vi "Linear Temperature Image.vi"() -> ()   [LabVIEW 2015]
doc: "An example of how you can get different types of images from the camera.\n\nNOTE: You must have ThermoVision installed to run this example."
uses:
  <userlib>/ThermoVision/ThermoVision Digital.llb/ThermoVision Digital ImageType.ctl
  <vilib>/Analysis/Matrix/NI_Matrix.lvlib
  <vilib>/Analysis/Matrix/Numeric/Conversions/Matrix To Array - RM.vi
  <userlib>/ThermoVision/ThermoVision.llb/Thermovision CameraTypes.ctl
  <userlib>/ThermoVision/ThermoVision.llb/ThermoVision DeviceTypes.ctl
  <userlib>/ThermoVision/ThermoVision.llb/ThermoVision CommunicationInterfaceType.ctl
  <userlib>/ThermoVision/ThermoVision Digital.llb/ThermoVision Digital ImageMode.ctl
panel:
  in  "Height Down":bool
  in  "Height Up":bool
  in  "Width Down":bool
  in  "Width Up":bool
  in  "Box Down":bool
  in  "Box Right":bool
  in  "Box Left":bool
  in  "Box Up":bool
  out "Camera":T1(plugin-control)
  out "Kelvin Multiplier":dbl=10.0
  out "Celsius":dbl
  out "Height":dbl=80.0
  out "Width":dbl=80.0
  out "Measure Box Y":dbl
  out "Measure Box X":dbl
  out "Average":dbl
  out "Total":dbl
  out "Image(U16)":u16[][](array[numeric])
  in  "Image Mode":T2=enum."Temperature (0.1K)"
  in  "Interface":T3=enum."UVC"
  in  "Device":T4=enum."USB video"
  in  "Camera Serial Number":string
  in  "CameraType":T5=enum."FLIR A615/A645/SC645/SC655"
  in  "error in (no error)":errorcluster
  in  "Stop":bool
  out "error out":errorcluster
  # "Note:\n Before running this VI\n 1. Select camera type supporting \n      linear temperature image (A-series)\n 2. Type camera serial number, if you \n     have more than one firewire camera\n     connected.\n 3. Run the VI\n 4. Press Stop button to terminate \n     VI-execution"
  # "Box Width"
  # "Box Position"
  # "Box Height"
  # "Pre-run settings"
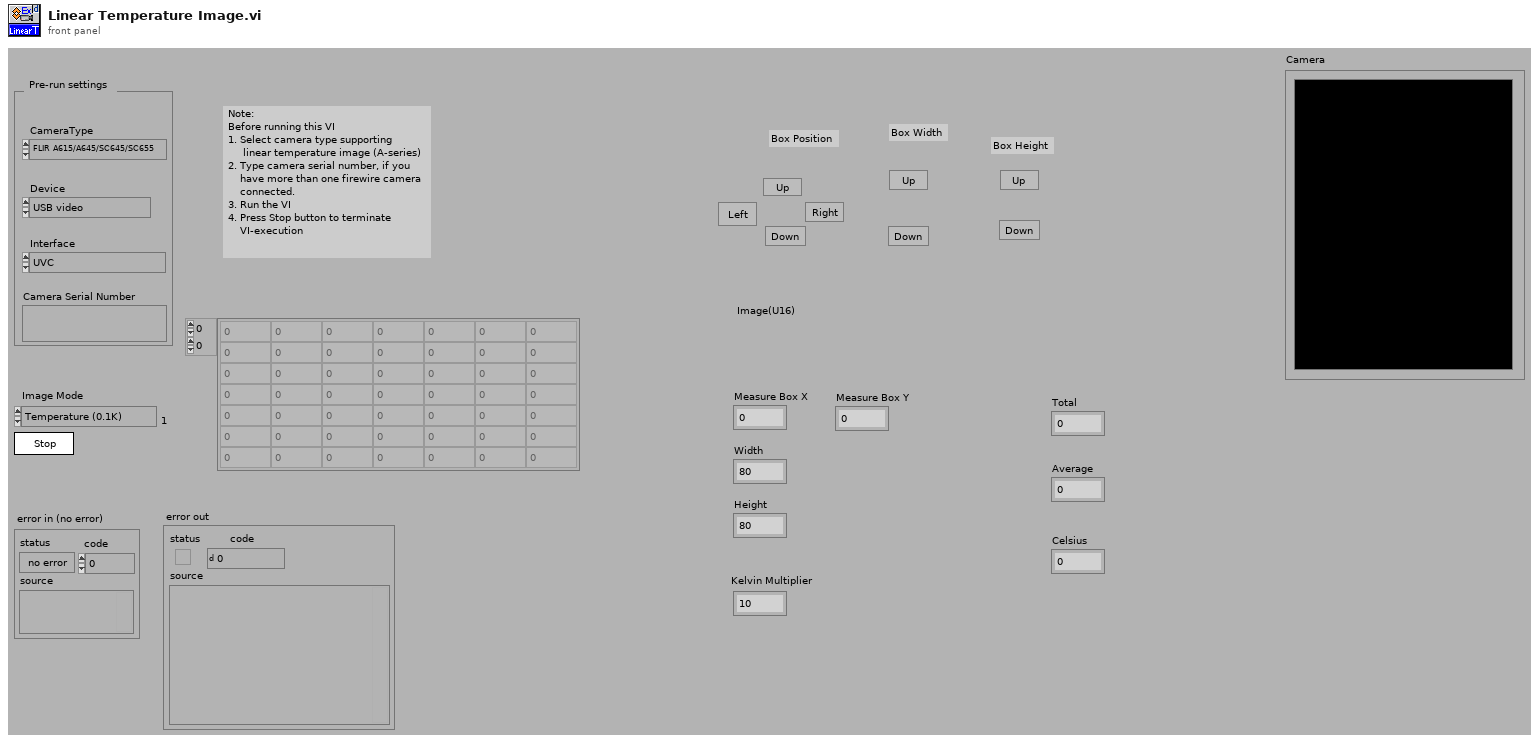
[diagram p1: front panel]
types:
  T1 = typedef "IMAQ Image.ctl" = refnum<image>
  T2 = typedef "ThermoVision Digital ImageMode.ctl" = enum16{"Signal", "Temperature (0.1K)", "Temperature (0.01K)"}
  T3 = typedef "ThermoVision CommunicationInterfaceType.ctl" = enum16{"File Only", "RS232", "TCP/IP(Ethernet)", "AV/C(FireWire)", "Gigabit Ethernet", "AXIS Video Server(Ethernet)", "UVC"}
  T4 = typedef "ThermoVision DeviceTypes.ctl" = enum16{"No Device", "FLIR PCCard", "ITEX IC-DIG 16", "Firewire 16-bit images", "Firewire 8-bit images", "Ethernet 16-bit images", "Ethernet 8-bit images", "IR-FlashLink", "iPort/GEV", "USB video"}
  T5 = typedef "Thermovision CameraTypes.ctl" = enum16{"ThermaCAM SC2000/SC3000", "THV 320/160", "ThermaCAM SC1000", "ThermaCAM S40/S45/S60/S65", "Thermovision A20/A40", "Cumulus SC4000/SC6000", "ThermaCAM SC640/SC660", "FLIR A320/A300/A310", "FLIR A325(A320G)/A315/SC305/SC325", "Indigo Merlin", "Indigo Phoenix", "Indigo Omega", "THV 1000", "THV 900", "FLIR GF320/GF309", "FLIR T-series", "FLIR A615/A645/SC645/SC655", "FLIR Exx series", "FLIR T620/T640/T420/T440"}
  T6 = enum16{"Internal Image Correction", "External Image Correction", "Auto Adjust", "Show Camera Info Dialog", "Show Device Status Dialog", "Reload Calibration(SC1000 only)"}
  T7 = enum16{"Unused0", "Unused1", "Unused2", "Unused3", "Unused4", "Unused5", "Unused6", "U16 Grayscale"}
  T8 = typedef "ThermoVision Digital ImageType.ctl" = enum16{"Raw", "Absolute", "Object", "Temperature", "Raw 8 bits"}
  T9 = typedef "Thermovision Object Reference.ctl" = refnum<k1>
  T10 = cluster{"Measure Box X":dbl, "Measure Box Y":dbl, dbl, dbl}
  T11 = typedef "LVPoint32TypeDef.ctl" = cluster{"Horizontal":i32, "Vertical":i32}
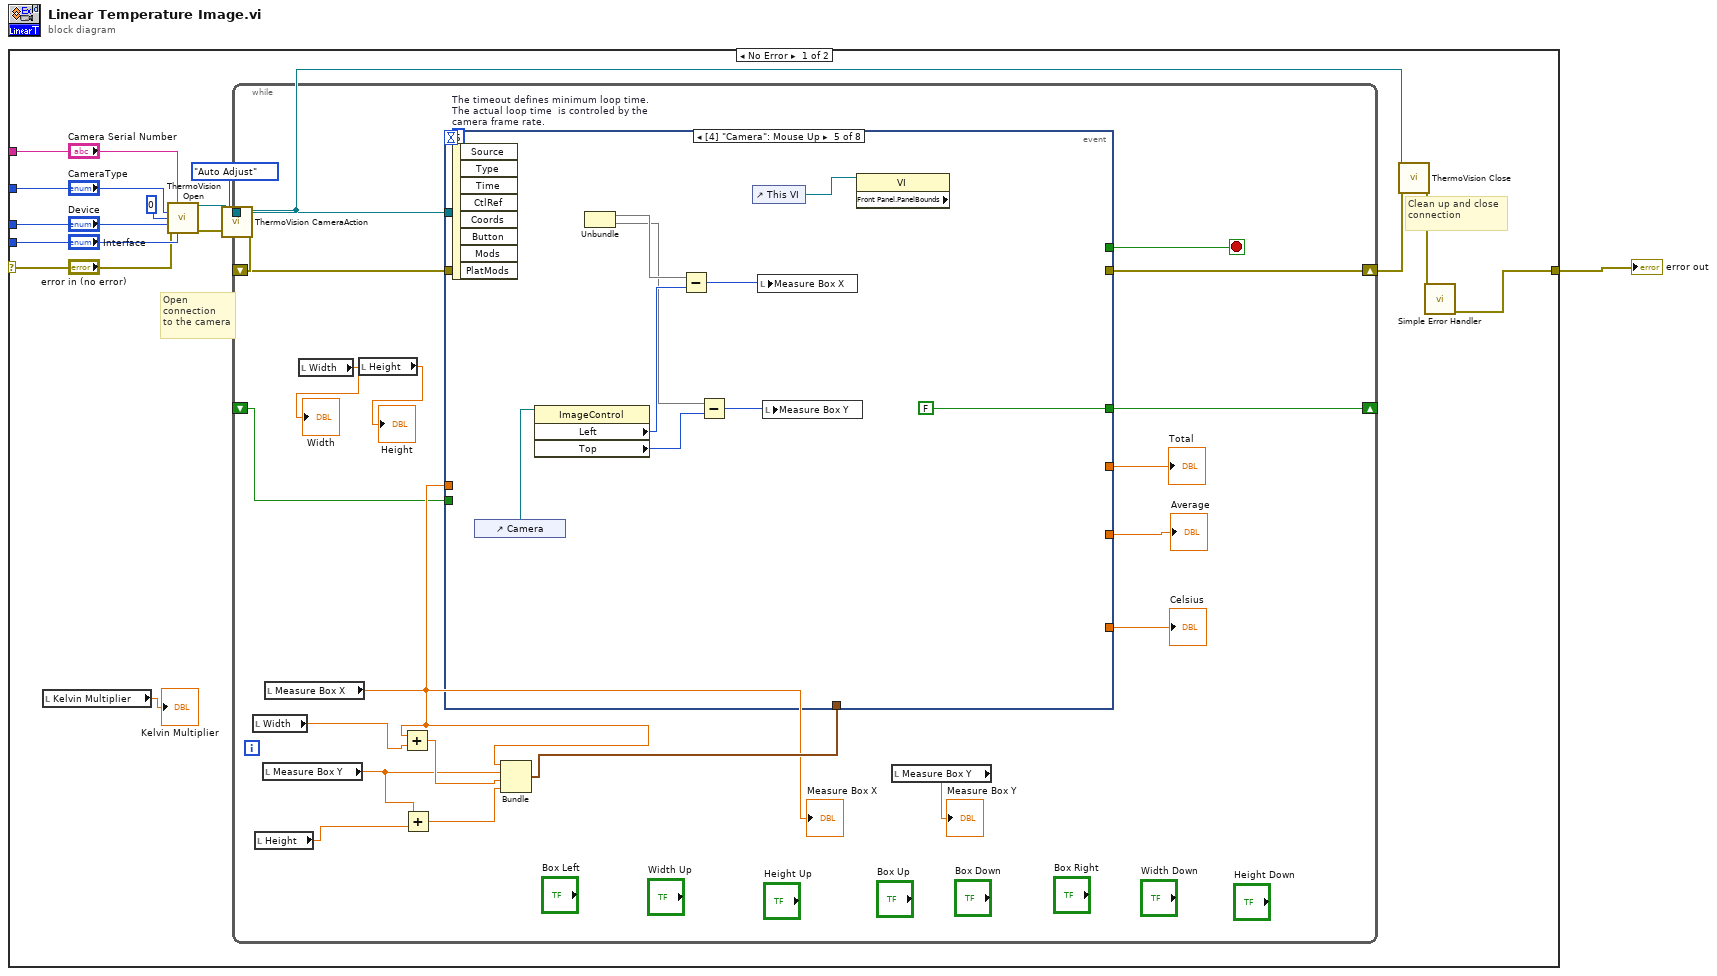
[diagram p0: block diagram]
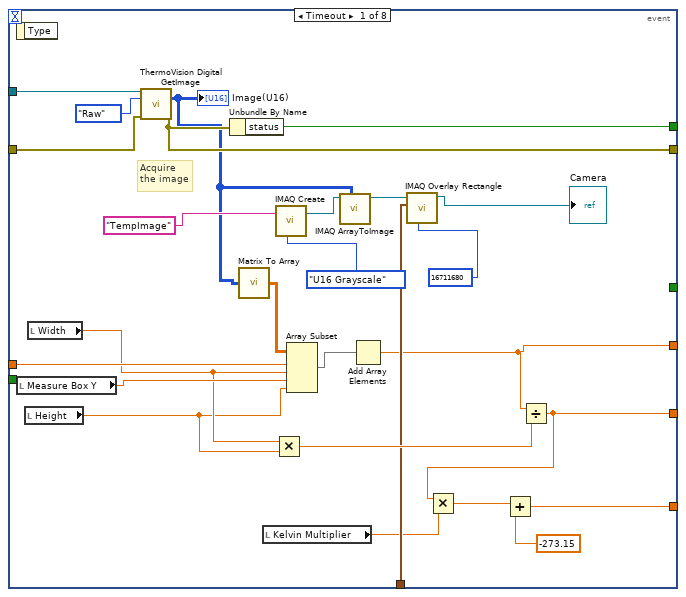
[diagram p2: hidden frame]
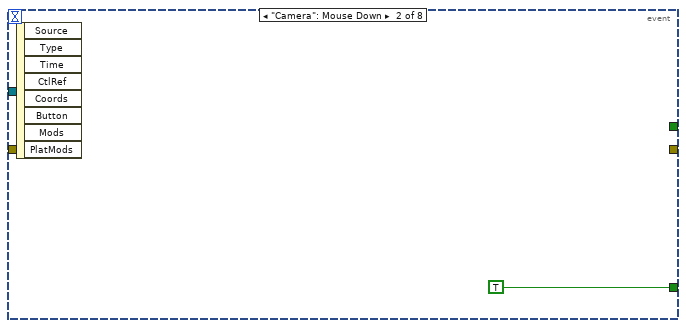
[diagram p3: hidden frame]
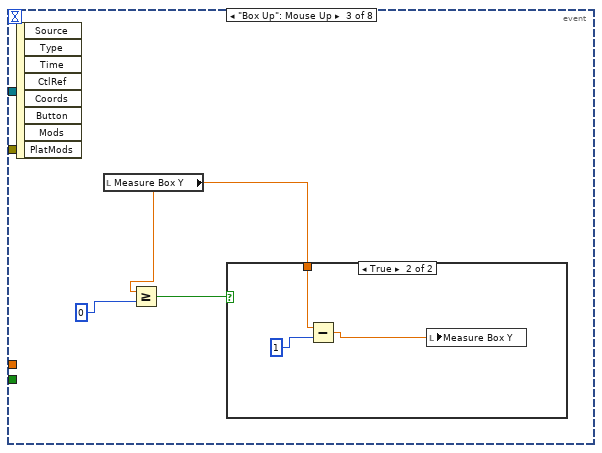
[diagram p4: hidden frame]
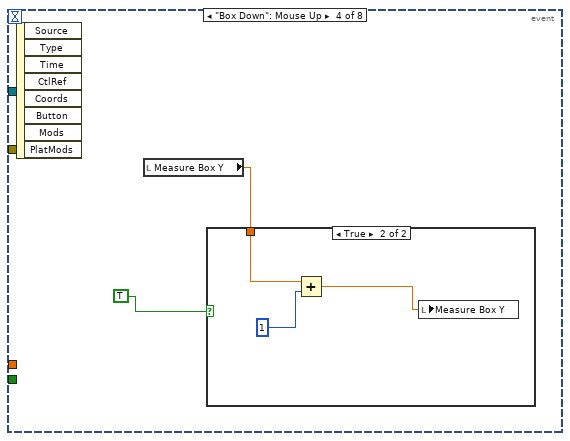
[diagram p6: hidden frame]
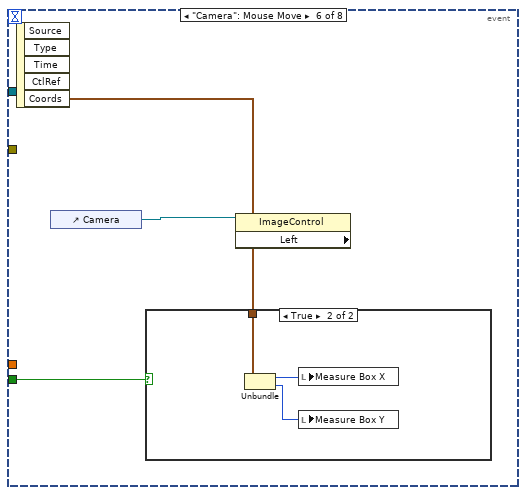
[diagram p8: hidden frame]
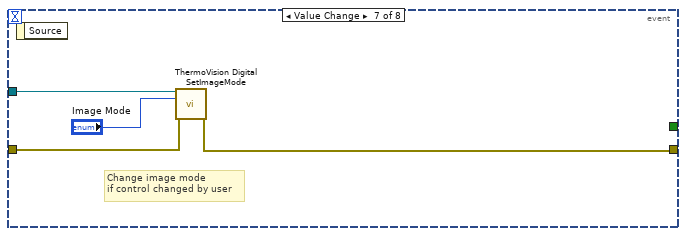
[diagram p10: hidden frame]
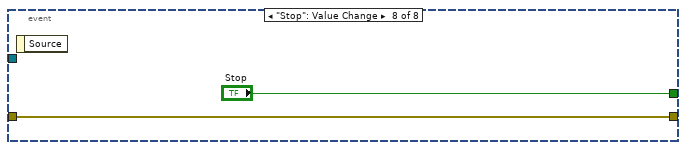
[diagram p11: hidden frame]
diagram:
  n1 = case shown="No Error" "error in (no error)" {
    selector: "error in (no error)" -> [w8 w101]
    tunnel: "CameraType" -> [w21 _]
    tunnel: [w19 w101] -> w5
    tunnel: "Camera Serial Number" -> [w17 _]
    tunnel: "Device" -> [w16 _]
    tunnel: "Interface" -> [w15 _]
    frame No Error {
      # "Open \nconnection\nto the camera"
      # "Clean up and close\nconnection"
      n2 = local read "Kelvin Multiplier"() -> (→"Kelvin Multiplier":dbl)
      n3 = call <userlib>:"ThermoVision Open.vi"("Server/SN"=w17, "CameraType"=w21, "Port"=i16 0, "Device"=w16, "error in (no error)"=w8, "Interface"=w15) -> ("reference"=w14:T9, "error out"=w12:errorcluster)  [unwired: 8 in]
      n4 = call <userlib>:"ThermoVision CameraAction.vi"("error in (no error)"=w12, "Action"=T6."Auto Adjust", "reference"=w14) -> ("error out"=w10:errorcluster, "duplicate reference"=w13:T9)  [unwired: 7 in]
      n5 = while {
        shift-right: [w40] -> w9
        shift-left: w10 -> [w39]
        tunnel: w13 -> [w41]
        shift-right: [w30] -> _
        shift-left: _ -> [w22]
        stop <- w37 stop-if-true
        w38 = 5  # The timeout defines minimum loop time.  The actual loop time  is controled by the camera frame rate.
        n6 = local read "Width"() -> (w24:dbl)
        n7 = local read "Height"() -> (w23:dbl)
        n8 = local read "Measure Box Y"() -> (w25:dbl)
        n9 = local read "Measure Box X"() -> (w29:dbl)
        "Measure Box X" <- w29
        n10 = local read "Width"() -> (→"Width":dbl)
        n11 = local read "Height"() -> (→"Height":dbl)
        n12 = Add(x=w29, y=w24) -> (x+y=w34:dbl)
        n13 = Add(x=w25, y=w23) -> (x+y=w36:dbl)
        n14 = Bundle("Measure Box X"=w29, "Measure Box Y"=w25, w34, w36) -> (w35:T10)  [unwired: 1 in]
        n15 = event shown="[4] \"Camera\": Mouse Up" {
          selector: _ -> [_ _ _ _ _ _ _ _]
          dyn-events: _ -> [_ _ _ _ _ _ _ _]
          timeout: w38 -> [_ _ _ _ _ _ _ _]
          tunnel: w39 -> [w63 _ _ _ _ _ w98 w99]
          tunnel: w41 -> [w66 _ _ _ _ _ w97 _]
          tunnel: [w65 _ _ _ _ _ w96 w99] -> w40
          tunnel: [w64 _ _ _ _ _ _ "Stop"] -> w37
          tunnel: w29 -> [w58 _ _ _ _ _ _ _]
          tunnel: w35 -> [w56 _ _ _ _ _ _ _]
          tunnel: [w49 _ _ _ _ _ _ _] -> w33
          tunnel: [w48 _ _ _ _ _ _ _] -> w32
          tunnel: [w47 _ _ _ _ _ _ _] -> w31
          tunnel: [_ TRUE _ _ FALSE _ _ _] -> w30
          tunnel: w22 -> [_ _ _ _ _ w91 _ _]
          event Timeout {
            # "Acquire\nthe image"
            n16 = event-data() -> ()  [unwired: 1 in, 1 out]
            n17 = local read "Measure Box Y"() -> (w45:dbl)
            n18 = local read "Height"() -> (w42:dbl)
            n19 = local read "Width"() -> (w43:dbl)
            n20 = call <userlib>:"ThermoVision Digital GetImage.vi"("reference"=w66, "ImageType"=ThermoVision_Digital_ImageType."Raw", "error in (no error)"=w63) -> ("Image(U16)"=w51:u16[][], "error out"=w65:errorcluster)  [unwired: 7 in, 4 out]
            "Image(U16)" <- w51
            n21 = Unbundle By Name(w65) -> ("status"=w64:bool)
            n22 = call-poly <vilib>:"Matrix To Array.vi"("Real Matrix"=w51) -> ("Real 2D Array"=w57:dbl[][])
            n23 = local read "Kelvin Multiplier"() -> (w44:dbl)
            n24 = Multiply(x=w43, y=w42) -> (x*y=w61:dbl)
            n25 = call "IMAQ Create"("Image Name"="TempImage", "Image Type"=T7."U16 Grayscale") -> ("New Image"=w54:T1)  [unwired: 3 in, 1 out]
            n26 = Array Subset(array=w57, index (row)=w58, length (row)=w43, index (col)=w45, length (col)=w42) -> (w62:dbl[][])
            n27 = call "IMAQ ArrayToImage"("Image Pixels (U16)"=w51, "Image"=w54) -> ("Image Out"=w55:T1)  [unwired: 8 in, 1 out]
            n28 = Add Array Elements(numeric array=w62) -> (sum=w48:dbl)
            n29 = call "IMAQ Overlay Rectangle"("Color"=16711680, "Rectangle"=w56, "Image"=w55) -> ("Image Out"=→"Camera":T1)  [unwired: 7 in, 1 out]
            n30 = Divide(x=w48, y=w61) -> (x/y=w47:dbl)
            n31 = Multiply(x=w47, y=w44) -> (x*y=w60:dbl)
            n32 = Add(x=w60, y=-273.15) -> (x+y=w49:dbl)
          }
          event "Camera": Mouse Down {
            n33 = event-data() -> ()  [unwired: 1 in, 8 out]
          }
          event "Box Up": Mouse Up {
            n34 = event-data() -> ()  [unwired: 1 in, 8 out]
            n35 = local read "Measure Box Y"() -> (w69:dbl)
            n36 = Greater Or Equal?(x=w69, y=0) -> (x >= y?=w70:bool)
            n37 = case shown="True" w70 {
              tunnel: w69 -> [_ w73]
              frame False {
              }
              frame True {
                n38 = Subtract(x=w73, y=1) -> (x-y=w74:dbl)
                n39 = local write "Measure Box Y"(w74) -> ()
              }
            }
          }
          event "Box Down": Mouse Up {
            n40 = event-data() -> ()  [unwired: 1 in, 8 out]
            n41 = local read "Measure Box Y"() -> (w75:dbl)
            n42 = case shown="True" TRUE {
              tunnel: w75 -> [_ w78]
              frame False {
              }
              frame True {
                n43 = Add(x=w78, y=1) -> (x+y=w77:dbl)
                n44 = local write "Measure Box Y"(w77) -> ()
              }
            }
          }
          event "Camera": Mouse Up {
            n45 = event-data() -> ()  [unwired: 1 in, 8 out]
            n46 = control-ref of="Camera"() -> (w81:refnum<vi>)
            n47 = property class="ImageControl"(reference=w81) -> ("Left"=w87:i32, "Top"=w83:i32)  [unwired: 1 in, 2 out]
            n48 = Unbundle() -> ("Horizontal"=w86, "Vertical"=w84)  [unwired: 1 in]
            n49 = Subtract(x=w86, y=w87) -> (x-y=w85:i32)
            n50 = Subtract(x=w84, y=w83) -> (x-y=w82:i32)
            n51 = control-ref of="This VI"() -> (w80:refnum<vi>)
            n52 = local write "Measure Box X"(w85) -> ()
            n53 = local write "Measure Box Y"(w82) -> ()
            n54 = property class="VI" props=["Front Panel.PanelBounds"](reference=w80) -> ()  [unwired: 1 in, 3 out]
          }
          event "Camera": Mouse Move {
            n55 = event-data() -> ("Coords"=w90:T11)  [unwired: 1 in, 4 out]
            n56 = control-ref of="Camera"() -> (w89:refnum<vi>)
            n57 = case shown="True" w91 {
              tunnel: w90 -> [_ w92]
              frame False {
              }
              frame True {
                n58 = Unbundle(w92) -> ("Horizontal"=w93:i32, "Vertical"=w94:i32)
                n59 = local write "Measure Box X"(w93) -> ()
                n60 = local write "Measure Box Y"(w94) -> ()
              }
            }
            n61 = property class="ImageControl" props=["Left"](reference=w89) -> ()  [unwired: 1 in, 3 out]
          }
          event Value Change {
            # "Change image mode\nif control changed by user"
            n62 = event-data() -> ()  [unwired: 1 in, 1 out]
            n63 = call <userlib>:"ThermoVision Digital SetImageMode.vi"("reference"=w97, "Image Mode"="Image Mode", "error in (no error)"=w98) -> ("error out"=w96:errorcluster)  [unwired: 11 in, 1 out]
          }
          event "Stop": Value Change {
            n64 = event-data() -> ()  [unwired: 1 in, 1 out]
          }
        }
        "Total" <- w32
        "Average" <- w31
        "Celsius" <- w33
        n65 = local read "Measure Box Y"() -> (→"Measure Box Y":dbl)
      }
      n66 = call <userlib>:"ThermoVision Close.vi"("reference"=w13, "error in (no error)"=w9) -> ("error out"=w20:errorcluster)  [unwired: 13 in]
      n67 = call <vilib>:"Simple Error Handler.vi"("error in (no error)"=w20) -> ("error out"=w19:errorcluster)  [unwired: 4 in, 4 out]
    }
    frame Error {
    }
  }
  "error out" <- w5
